vi "TPOSE.vi"() -> ()   [LabVIEW 2018]
doc: "Manually blink and LED attached to a digital output channel of a LINX device by clicking and LED control in LabVIEW."
uses:
  <vilib>/MakerHub/LINX/Public/Peripherals/Digital/Digital Write 1 Chan.vi
  <vilib>/MakerHub/LINX/Public/Peripherals/Analog/Analog Read 1 Chan.vi
  <vilib>/MakerHub/LINX/Public/Peripherals/Digital/Digital Write N Chans.vi
  <vilib>/MakerHub/LINX/Public/Peripherals/Analog/Analog Read N Chans.vi
  <vilib>/MakerHub/LINX/Private/Local IO/LinxDigitalWrite.vi
  <vilib>/MakerHub/LINX/Public/Utilities/Check Channel.vi
  <vilib>/MakerHub/LINX/Private/Local IO/LinxAnalogRead.vi
  <vilib>/MakerHub/LINX/Public/Utilities/Open Serial.vi
  <vilib>/MakerHub/LINX/Private/Utilties/Generate Error.vi
  <vilib>/MakerHub/LINX/LMH-LINX.lvlib
panel:
  in  "CUCHILLA ELECTRICA 2":bool
  out "VENTILADOR":bool
  in  "CUCHILLA ELECTRICA":bool
  in  "Limite de Temperatura Bajo":u32(knob) scale=0.0..70.0
  in  "Salida Digital (Calentador)":u8=13
  out "s":bool
  in  "Modo de Control":string(combo)
  in  "Salida Digital (Ventilador)":u8=13
  in  "Limite de Temperatura Alta":u32(knob) scale=0.0..70.0
  out "Waveform Chart 2":T1(graph)
  in  "Salida Analogica (Sensor)":u8
  out "Temperatura":dbl
  out "Termometro":dbl(slide) scale=0.0..100.0
  out "Loop Rate (Hz)":u32
  in  "LED Value":bool
  in  "Salida Digital (Foco)":u8=13
  in  "Puerto Serial":refnum<visa-resource-name>
  in  "Stop Button":bool
  # "Conexiones"
  # "Ventilador"
  # "Calentador"
  # "Prueba de Conexion"
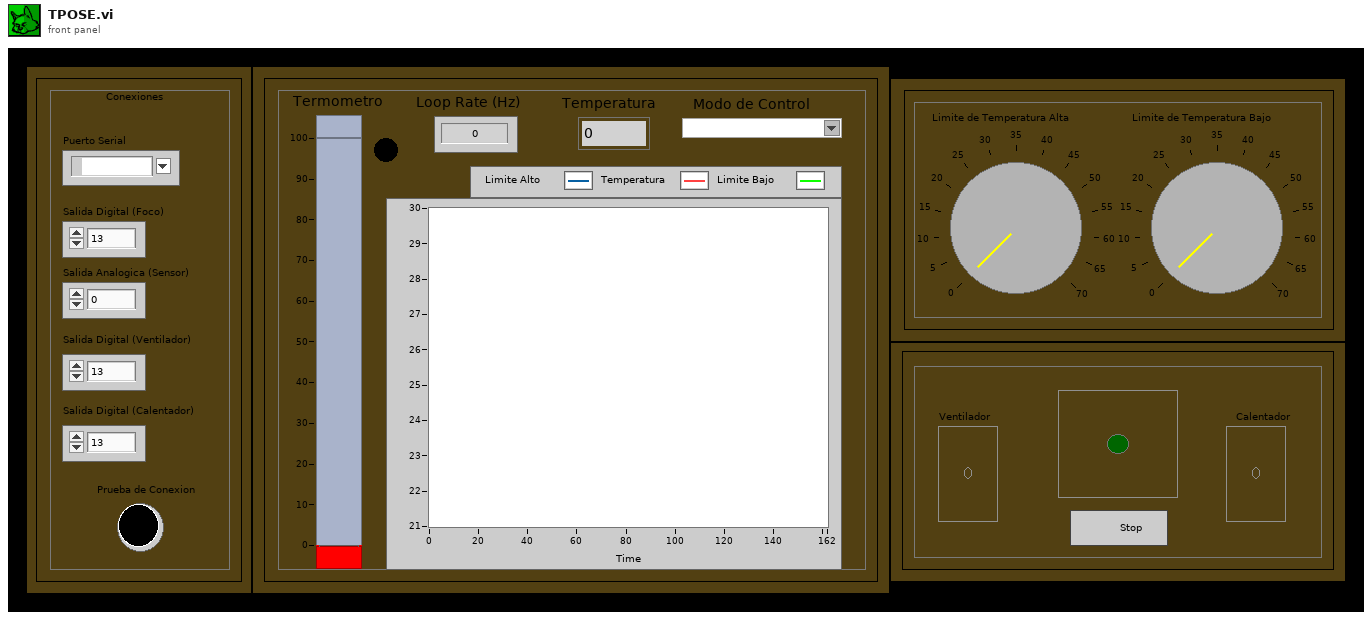
[diagram p1: front panel]
types:
  T1 = cluster{"Limite de Temperatura Alta":u32, dbl, "Limite de Temperatura Alta 2":u32}
  T2 = typedef "LMH-LINX.lvlib/LINX Ref.ctl" = cluster{"IO":T3, "Interface":T4, "LINX Device Config":T5}
  T3 = typedef "LMH-LINX.lvlib/Platform.ctl" = enum16{"Remote", "Local"}
  T4 = typedef "LMH-LINX.lvlib/Interface.ctl" = enum16{"Serial", "TCP"}
  T5 = typedef "LMH-LINX.lvlib/Device.lvlib/LINX Device Config.ctl" = cluster{"Interface":T4, "COM Port":refnum<visa-resource-name>, "TCP Configuration":T6, "Device Family":u8, "Device ID":u8, "Device Name":string, "TCP Ref":refnum<k5>, "Channels":T7}
  T6 = typedef "LMH-LINX.lvlib/Device.lvlib/TCP Config.ctl" = cluster{"IP Address":string, "Port":u16}
  T7 = typedef "LMH-LINX.lvlib/Channels.ctl" = cluster{"DI":u8[], "DO":u8[], "AI":u8[], "AO":u8[], "PWM":u8[], "QE":u8[], "UART":u8[], "I2C 2":u8[], "SPI":u8[], "CAN":u8[], "Servo":u8[], "AI Ref (V)":dbl, "AI Resolution (Bits)":u8, "AO Ref (V)":dbl, "AO Resolution (Bits)":u8}
  T8 = cluster{"Limite de Temperatura Alta":u32, dbl, "Limite de Temperatura Bajo":u32}
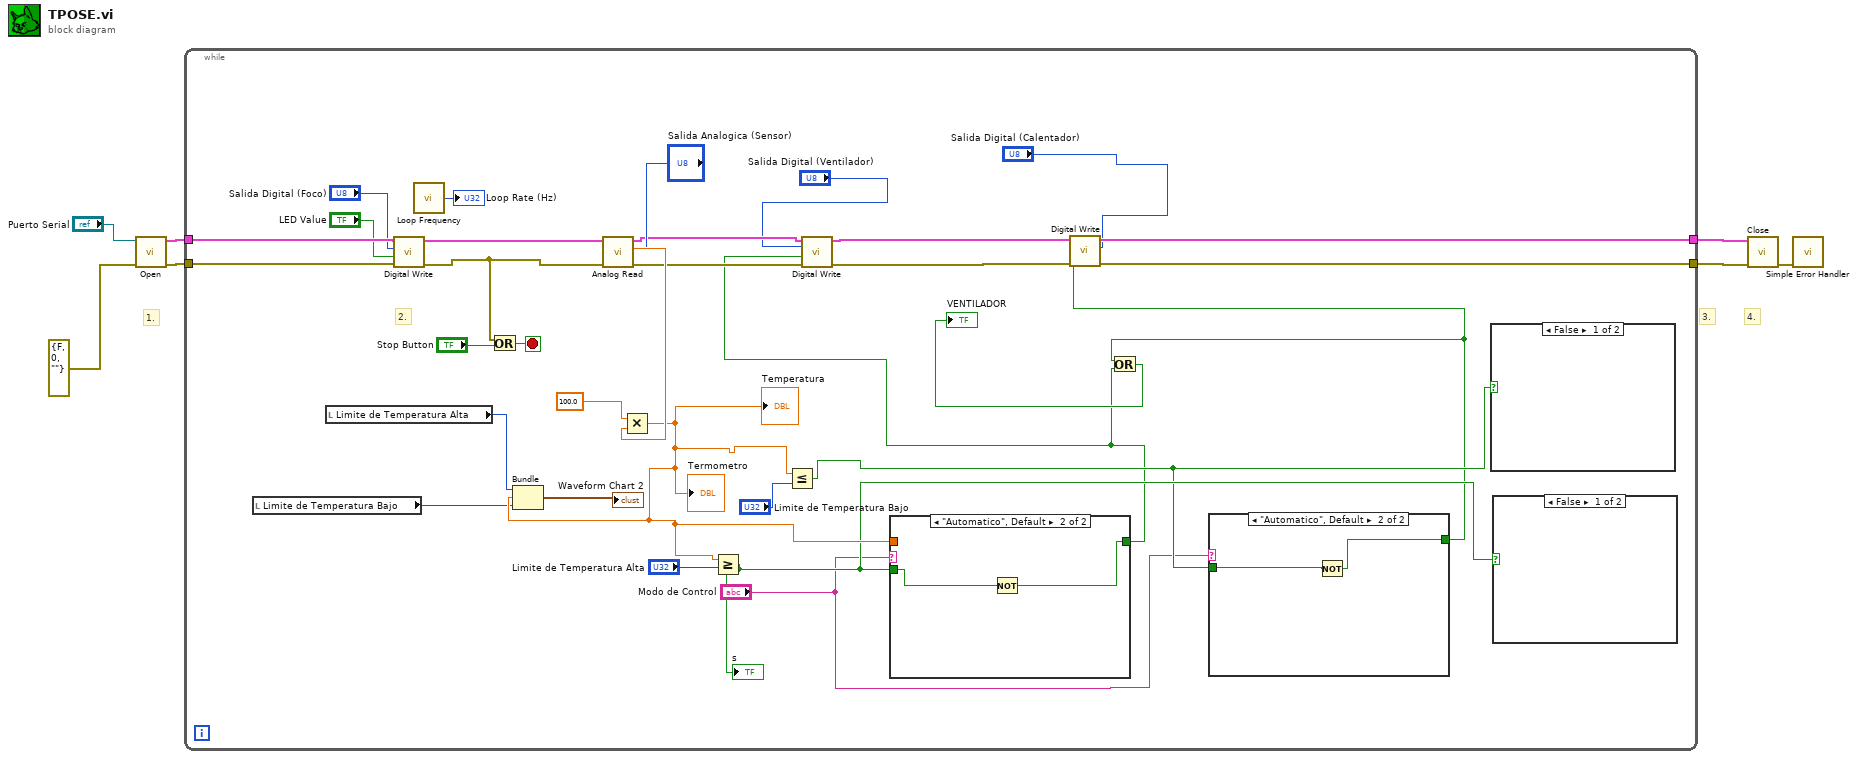
[diagram p0: block diagram]
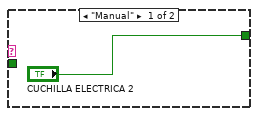
[diagram p2: hidden frame]
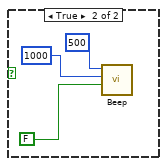
[diagram p3: hidden frame]
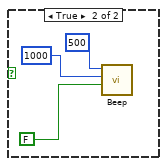
[diagram p4: hidden frame]
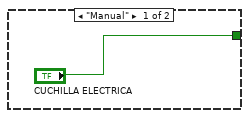
[diagram p5: hidden frame]
diagram:
  # "4."
  # "3."
  # "1."
  n1 = call-poly <vilib>:"Open.vi"("Error In"=errorcluster {"status"=FALSE, "code"=0, "source"=""}, "Serial Port"="Puerto Serial") -> ("Error Out"=w3:errorcluster, "LINX Resource"=w7:T2)  [unwired: 7 in, 1 out]
  n2 = while {
    tunnel: w7 -> [w37]
    tunnel: w3 -> [w28]
    tunnel: [w21] -> w2
    tunnel: [w20] -> w1
    stop <- w39 stop-if-true
    # "2."
    n3 = local read "Limite de Temperatura Bajo"() -> (w16:u32)
    n4 = local read "Limite de Temperatura Alta"() -> (w24:u32)
    n5 = call-poly <vilib>:"Digital Write.vi"("Error In"=w28, "Output Value"="LED Value", "DO Channel"="Salida Digital (Foco)", "LINX Resource"=w37) -> ("Error Out"=w32:errorcluster, "LINX Resource"=w33:T2)  [unwired: 6 in]
    n6 = call <vilib>:"Loop Frequency.vi"() -> ("Loop Rate (Hz)"=→"Loop Rate (Hz)":u32)
    n7 = Or(x=w32, y="Stop Button") -> (x .or. y?=w39:bool)
    n8 = call-poly <vilib>:"Analog Read.vi"("Error In"=w32, "Analog Channel"="Salida Analogica (Sensor)", "LINX Resource"=w33) -> ("Error Out"=w26:errorcluster, "Voltage"=w30:dbl, "LINX Resource"=w27:T2)  [unwired: 5 in, 1 out]
    n9 = Multiply(x=100.0, y=w30) -> (x*y=w18:dbl)
    "Termometro" <- w18
    "Temperatura" <- w18
    n10 = Bundle("Limite de Temperatura Alta"=w24, w18, "Limite de Temperatura Bajo"=w16) -> (→"Waveform Chart 2":T8)  [unwired: 1 in]
    n11 = Greater Or Equal?(x=w18, y="Limite de Temperatura Alta") -> (x >= y?=w13:bool)
    "s" <- w13
    n12 = Less Or Equal?(x=w18, y="Limite de Temperatura Bajo") -> (x <= y?=w12:bool)
    n13 = case shown="\"Automatico\", Default" "Modo de Control" {
      tunnel: ["CUCHILLA ELECTRICA" w50] -> w8
      tunnel: w18 -> [_ _]
      tunnel: w13 -> [_ w51]
      frame "Manual" {
      }
      frame "Automatico", Default {
        n14 = Not(x=w51) -> (.not. x?=w50:bool)
      }
    }
    n15 = call-poly <vilib>:"Digital Write.vi"("Error In"=w26, "Output Value"=w8, "DO Channel"="Salida Digital (Ventilador)", "LINX Resource"=w27) -> ("Error Out"=w22:errorcluster, "LINX Resource"=w23:T2)  [unwired: 6 in]
    n16 = case shown="\"Automatico\", Default" "Modo de Control" {
      tunnel: ["CUCHILLA ELECTRICA 2" w41] -> w9
      tunnel: w12 -> [_ w42]
      frame "Manual" {
      }
      frame "Automatico", Default {
        n17 = Not(x=w42) -> (.not. x?=w41:bool)
      }
    }
    n18 = call-poly <vilib>:"Digital Write.vi"("Error In"=w22, "Output Value"=w9, "DO Channel"="Salida Digital (Calentador)", "LINX Resource"=w23) -> ("Error Out"=w20:errorcluster, "LINX Resource"=w21:T2)  [unwired: 6 in]
    n19 = Or(x=w9, y=w8) -> (x .or. y?=→"VENTILADOR":bool)
    n20 = case shown="False" w12 {
      frame False {
      }
      frame True {
        n21 = call <vilib>:"Beep.vi"("use system alert? (T)"=FALSE, "duration (msec)"=u32 1000, "frequency (Hz)"=u32 500) -> ()  [unwired: 9 in]
      }
    }
    n22 = case shown="False" w13 {
      frame False {
      }
      frame True {
        n23 = call <vilib>:"Beep.vi"("use system alert? (T)"=FALSE, "duration (msec)"=u32 1000, "frequency (Hz)"=u32 500) -> ()  [unwired: 9 in]
      }
    }
  }
  n24 = call <vilib>:"Close.vi"("Error In"=w1, "LINX Resource"=w2) -> ("Error Out"=w5:errorcluster)  [unwired: 9 in]
  n25 = call <vilib>:"Simple Error Handler.vi"("error in (no error)"=w5) -> ()  [unwired: 4 in, 5 out]
